vi "Initialize.vi"(8 "error in":errorcluster, 11 "Plugin in":refnum<class "CSV Export.lvclass">) -> (0 "error out":errorcluster, 3 "Plugin out":refnum<class "CSV Export.lvclass">)   [LabVIEW 2022 SP3, in "CSV Export.lvlib" / "CSV Export.lvclass"]
uses:
  CSV Export.lvclass
  C:/Program Files/National Instruments/LabVIEW 2022/vi.lib/FlexLogger/SDK/PluginSDK.lvlibp/PEFClasses/SDK/Plugin/Plugin.lvclass
  C:/Program Files/National Instruments/LabVIEW 2022/vi.lib/FlexLogger/SDK/PluginSDK.lvlibp/PEFClasses/SDK/Processing Element/Processing Element.lvclass
  <vilib>/FlexLogger/SDK/PluginSDK.lvlibp/PEFClasses/SDK/Processing Element/Timing Parameters.ctl
  <vilib>/FlexLogger/SDK/PluginSDK.lvlibp/PEFClasses/SDK/Processing Element/Timing Method.ctl
  Controls/CSV Export Settings.ctl
  CSV Export.lvclass/CSV Export.ctl
  <vilib>/FlexLogger/SDK/PluginSDK.lvlibp/PEFClasses/SDK/Plugin/ParameterAccess/Write Command.vi
  <vilib>/FlexLogger/SDK/PluginSDK.lvlibp/PEFClasses/SDK/Processing Element/Read System Interface.vi
  <vilib>/FlexLogger/SDK/PluginSDK.lvlibp/PEFClasses/SDK/Processing Element/Read Alias.vi
  Global.vi
  <vilib>/FlexLogger/SDK/PluginSDK.lvlibp/PEFClasses/SDK/Plugin/Plugin.lvclass
  <vilib>/FlexLogger/SDK/PluginSDK.lvlibp/PEFClasses/SDK/System Interface/System Interface.lvclass
  <vilib>/FlexLogger/SDK/PluginSDK.lvlibp/PEFClasses/SDK/Processing Element/Processing Element.lvclass
  C:/Users/bbuchana/Documents/LabVIEW Projects/FlexLogger IO Plug-ins/CSV Export/CSV Export.lvclass
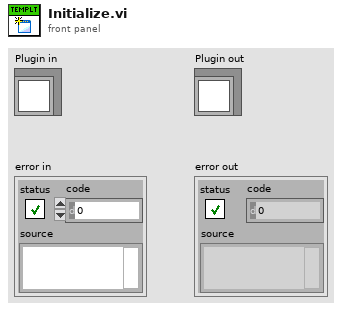
[diagram p1: front panel]
types:
  T1 = typedef "CSV Export.lvlib/CSV Export.lvclass/CSV Export Settings.ctl" = cluster{"Log Stats":bool, "Time Format":string, "Resampled":bool, "Resampled Rate":dbl, "Digits of Precision":u32, "Relative Time":bool, "Log Units":bool, "Log Properties":bool}
  T2 = typedef "PluginSDK.lvlibp/Processing Element.lvclass/Timing Parameters.ctl" = cluster{"Timing Method":T3, "Timing Period (ms)":i32}
  T3 = typedef "PluginSDK.lvlibp/Processing Element.lvclass/Timing Method.ctl" = enum16{"Periodic", "Immediate", "On Data Ready", "Triggered"}
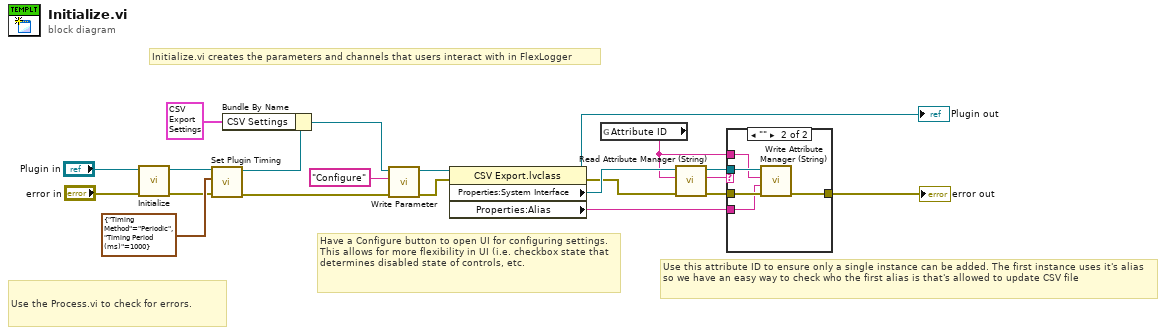
[diagram p0: block diagram]
diagram:
  # "Use this attribute ID to ensure only a single instance can be added. The first instance uses it's alias so we have an easy way to check who the first alias is that's allowed to update CSV file"
  # "Have a Configure button to open UI for configuring settings. This allows for more flexibility in UI (i.e. checkbox state that determines disabled state of controls, etc."
  # "Use the Process.vi to check for errors."
  # "Initialize.vi creates the parameters and channels that users interact with in FlexLogger"
  n1 = call-parent "Initialize.vi"("error in (no error)"="error in", "Plugin in"="Plugin in") -> ("error out"=w17:errorcluster, "Plugin out"=w16:refnum<class "CSV Export.lvclass">)  [unwired: 8 in]
  n2 = call <vilib>:"Set Plugin Timing.vi"("error in (no error)"=w17, "Timing Parameters"=T2 {"Timing Method"=enum."Periodic", "Timing Period (ms)"=1000}, "Plugin in"=w16) -> ("error out"=w15:errorcluster, "Plugin out"=w14:refnum<class "CSV Export.lvclass">)  [unwired: 7 in]
  n3 = Bundle By Name(cluster=w14, "CSV Settings"=T1 {"Log Stats"=TRUE, "Time Format"="%H:%M:%S%3u", "Resampled"=TRUE, "Resampled Rate"=100.0, "Digits of Precision"=3, "Relative Time"=TRUE, "Log Units"=FALSE, "Log Properties"=FALSE}) -> (w13:refnum<class "CSV Export.lvclass">)
  n4 = call-poly <vilib>:"Write Parameter.vi"("error in (no error)"=w15, "Name"="Configure", "Plugin in"=w13) -> ("error out"=w11:errorcluster, "Plugin out"=w12:refnum<class "CSV Export.lvclass">)  [unwired: 7 in]
  n5 = property class="CSV Export.lvclass"(reference=w12, error in=w11) -> (reference out=→"Plugin out":refnum<class "CSV Export.lvclass">, error out=w9:errorcluster, "Properties:System Interface"=w10:refnum<class "System Interface.lvclass">, "Properties:Alias"=w2:string)
  n6 = global read "Global.vi" "Attribute ID"() -> (w5:string)
  n7 = call-dynamic "Read Attribute Manager (String).vi"("error in (no error)"=w9, "Attribute ID"=w5, "System Interface in"=w10) -> ("error out"=w7:errorcluster, "Attrib Val"=w3:string, "System Interface out"=w8:refnum<class "System Interface.lvclass">)  [unwired: 5 in, 1 out]
  n8 = case shown="\"\"" w3 {
    tunnel: w8 -> [_ w27]
    tunnel: w7 -> [w22 w26]
    tunnel: w2 -> [_ w24]
    tunnel: w5 -> [_ w25]
    tunnel: [w22 w23] -> w4
    frame Default {
      # "An instance already exists. Let Process.vi return error"
    }
    frame "" {
      n9 = call-dynamic "Write Attribute Manager (String).vi"("error in (no error)"=w26, "Attribute Value"=w24, "Attribute ID"=w25, "System Interface in"=w27) -> ("error out"=w23:errorcluster)  [unwired: 5 in, 2 out]
    }
  }
  "error out" <- w4
